vi "CRYCheck Amplitude.vi"(9 "Sens Value":dbl, 10 "Vp Out":dbl=1.0 min=0.1 step=0.01 format="%.2f", 11 "Stimulus max value":sgl) -> (3 "Overflow":bool)   [LabVIEW 2013]
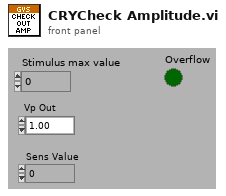
[diagram p1: front panel]
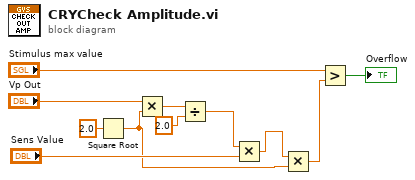
[diagram p0: block diagram]
diagram:
  n1 = Square Root(x=2.0) -> (sqrt(x)=w3:dbl)
  n2 = Multiply(x="Vp Out", y=w3) -> (x*y=w6:dbl)
  n3 = Divide(x=w6, y=2.0) -> (x/y=w5:dbl)
  n4 = Multiply(x=w5, y="Sens Value") -> (x*y=w4:dbl)
  n5 = Multiply(x=w4, y=w3) -> (x*y=w1:dbl)
  n6 = Greater?(x="Stimulus max value", y=w1) -> (0:→"Overflow":bool)
